vi "Host Stream Engine.vi"(8 "error in (no error)":errorcluster, 9 "Sort By ID":bool, 10 "Pause":bool, 11 "Cmd Q":refnum<queue>) -> (0 "error out":errorcluster, 1 "Exit":bool, 3 "Stream":T1)   [LabVIEW 2019, in "CAN Streaming Support Workspace Shared.lvlib"]
uses:
  CAN Streaming Support Workspace Shared.lvlib
  Types/Host Stream API Data.ctl
  Types/Host Stream API Queue Type.ctl
  Types/Host Stream API Queue Cmd.ctl
  Types/Host Stream API Engine State.ctl
  Process CAN Data.vi
  Process CAN State.vi
  <userlib>/_OpenG.lib/array/array.llb/Sort Array__ogtk.vi
  <userlib>/_OpenG.lib/array/array.llb/Sort 2D Array (String)__ogtk.vi
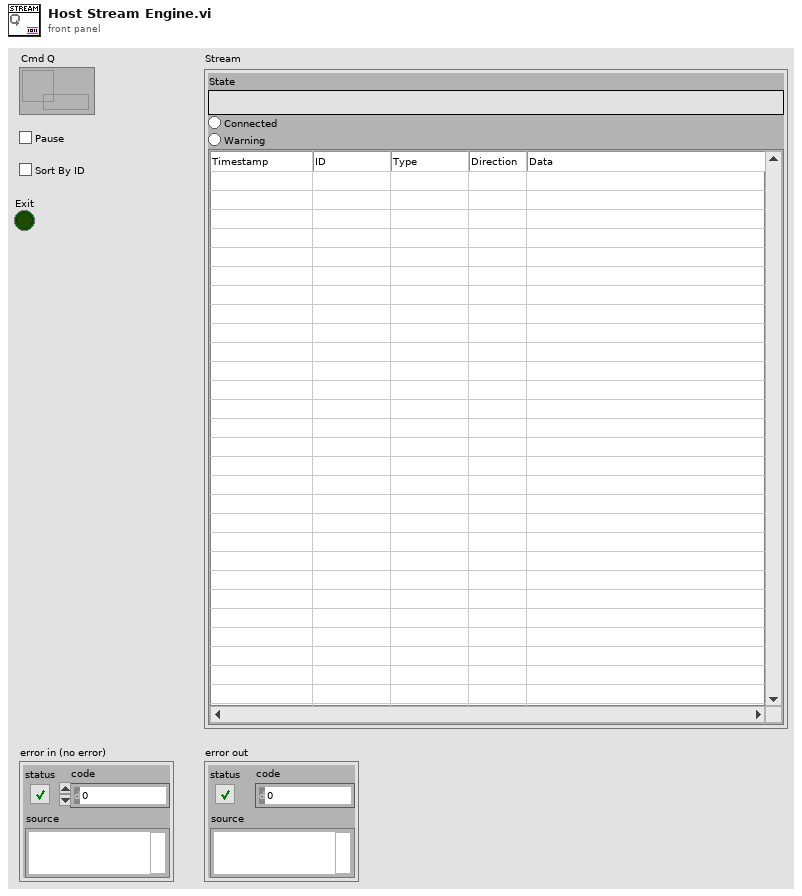
[diagram p1: front panel]
types:
  T1 = typedef "CAN Streaming Support Workspace Shared.lvlib/Host Stream API Data.ctl" = cluster{"State":string, "Connected":bool, "Warning":bool, "Table":string[][]}
  T2 = typedef "CAN Streaming Support Workspace Shared.lvlib/Host Stream API Engine State.ctl" = enum8{"Wait", "Start Stream", "Read Stream", "Stop Stream", "Exit"}
  T3 = typedef "CAN Streaming Support Workspace Shared.lvlib/Host Stream API Queue Type.ctl" = cluster{"Cmd":T4, "Target IP Address":string, "Addon":string}
  T4 = typedef "CAN Streaming Support Workspace Shared.lvlib/Host Stream API Queue Cmd.ctl" = enum8{"Start Stream", "Stop Stream", "Exit"}
  T5 = typedef "CAN Streaming Support Workspace Shared.lvlib/Host Stream API Refs.ctl" = cluster{"Target IP Address":string, "Addon":string, "Stream Ref":refnum<k21>}
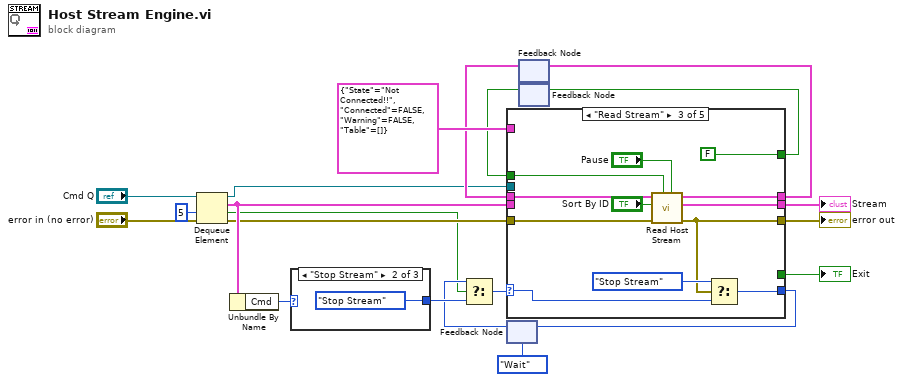
[diagram p0: block diagram]
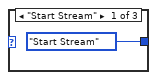
[diagram p2: hidden frame]
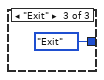
[diagram p3: hidden frame]
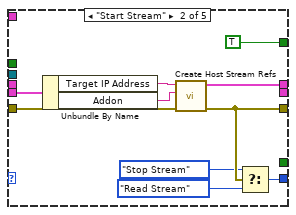
[diagram p5: hidden frame]
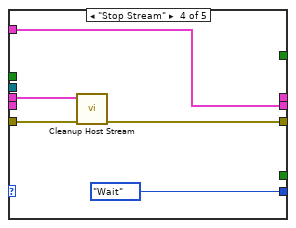
[diagram p6: hidden frame]
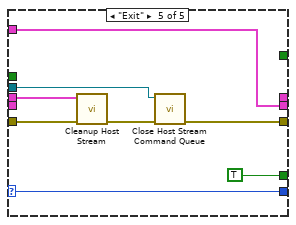
[diagram p7: hidden frame]
diagram:
  n1 = Dequeue Element(queue="Cmd Q", timeout in ms (-1)=5, error in (no error)="error in (no error)") -> (queue out=w1:refnum<queue>, element=w11:T3, timed out?=w4:bool, error out=w9:errorcluster)
  n2 = Unbundle By Name(w11) -> ("Cmd"=w12:T4)
  n3 = case shown="\"Stop Stream\"" w12 {
    tunnel: [Host_Stream_API_Engine_State."Start Stream" Host_Stream_API_Engine_State."Stop Stream" Host_Stream_API_Engine_State."Exit"] -> w13
    frame "Start Stream" {
    }
    frame "Stop Stream" {
    }
    frame "Exit" {
    }
  }
  n4 = feedback #1(Host_Stream_API_Engine_State."Wait") -> (w7:T2)
  n5 = Select(t=w7, s=w4, f=w13) -> (s? t:f=w8:T2)
  n6 = feedback #2() -> (w15:T5)  [unwired: 1 in]
  n7 = feedback #3() -> (w17:bool)  [unwired: 1 in]
  n8 = case shown="\"Read Stream\"" w8 {
    selector: w8 -> [w25 _ w39 _ w59]
    tunnel: w9 -> [w27 w37 w49 w54 w62]
    tunnel: w11 -> [_ w36 _ _ _]
    tunnel: [w27 w31 w40 w53 w56] -> w21
    tunnel: [_ w33 w47 _ _] -> w14
    tunnel: w15 -> [_ _ w48 w52 w61]
    tunnel: [w26 _ w46 w51 w60] -> w19
    tunnel: [_ TRUE FALSE _ _] -> w16
    tunnel: w17 -> [_ _ w45 _ _]
    tunnel: T1 {"State"="Not Connected!!", "Connected"=FALSE, "Warning"=FALSE, "Table"=[]} ("Stream") -> [w26 _ _ w51 w60]
    tunnel: [w25 w28 w38 Host_Stream_API_Engine_State."Wait" w59] -> w20
    tunnel: [_ _ _ _ TRUE] -> w2
    tunnel: w1 -> [_ _ _ _ w55]
    frame "Wait", Default {
    }
    frame "Start Stream" {
      n9 = Unbundle By Name(w36) -> ("Target IP Address"=w35:string, "Addon"=w34:string)
      n10 = call "Create Host Stream Refs.vi"("error in (no error)"=w37, "Addon"=w34, "Target IP Address"=w35) -> ("error out"=w31:errorcluster, "Refs"=w33:T5)  [unwired: 7 in]
      n11 = Select(t=Host_Stream_API_Engine_State."Stop Stream", s=w31, f=Host_Stream_API_Engine_State."Read Stream") -> (s? t:f=w28:T2)
    }
    frame "Read Stream" {
      n12 = call "Read Host Stream.vi"("Pause"="Pause", "Init?"=w45, "error in (no error)"=w49, "Sort By ID"="Sort By ID", "Refs in"=w48) -> ("error out"=w40:errorcluster, "Stream"=w46:T1, "Refs out"=w47:T5)  [unwired: 4 in]
      n13 = Select(t=Host_Stream_API_Engine_State."Stop Stream", s=w40, f=w39) -> (s? t:f=w38:T2)
    }
    frame "Stop Stream" {
      n14 = call "Cleanup Host Stream.vi"("error in (no error)"=w54, "Refs"=w52) -> ("error out"=w53:errorcluster)  [unwired: 9 in]
    }
    frame "Exit" {
      n15 = call "Cleanup Host Stream.vi"("error in (no error)"=w62, "Refs"=w61) -> ("error out"=w57:errorcluster)  [unwired: 9 in]
      n16 = call "Close Host Stream Command Queue.vi"("error in (no error)"=w57, "Cmd Q"=w55) -> ("error out"=w56:errorcluster)  [unwired: 9 in]
    }
  }
  "Stream" <- w19
  "error out" <- w21
  "Exit" <- w2
  n17 = feedback-in #1(w20) -> ()
  n18 = feedback-in #2(w14) -> ()
  n19 = feedback-in #3(w16) -> ()
